vi "SnpxIsConnected.vi"(10 "Snpx":refnum<k24>, 11 "error in":errorcluster) -> (2 "Connected":bool, 3 "error out":errorcluster)   [LabVIEW 2023, in "UnderAutomation.Fanuc.lvlib"]
uses:
  UnderAutomation.Fanuc.lvlib
  C:/Users/fg/Documents/Fanuc.vi/LabVIEW_2024/UnderAutomation.Fanuc/lib/UnderAutomation.Fanuc.dll
  LabVIEW_2024/UnderAutomation.Fanuc/lib/UnderAutomation.Fanuc.dll
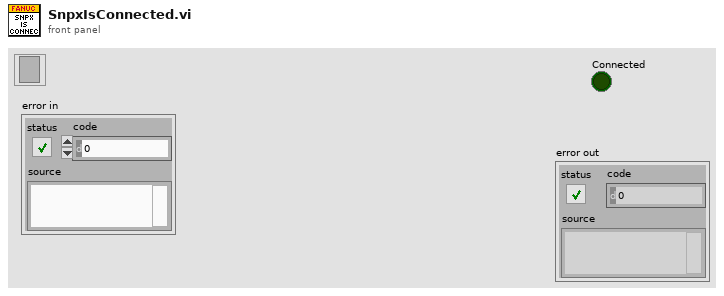
[diagram p1: front panel]
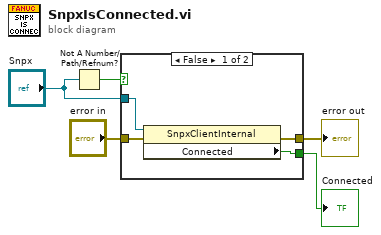
[diagram p0: block diagram]
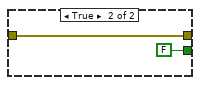
[diagram p2: hidden frame]
diagram:
  n1 = Not A Number/Path/Refnum?(number/path/refnum="Snpx") -> (NaN/Path/Refnum?=w5:bool)
  n2 = case shown="False" w5 {
    tunnel: "Snpx" -> [w9 _]
    tunnel: "error in" -> [w8 w11]
    tunnel: [w7 w11] -> w3
    tunnel: [w6 FALSE ("Connected")] -> w2
    frame False {
      n3 = property class="SnpxClientInternal"(reference=w9, error in=w8) -> (error out=w7:errorcluster, "Connected"=w6:bool)  [unwired: 1 out]
    }
    frame True {
    }
  }
  "error out" <- w3
  "Connected" <- w2
